vi "RM.set listbox size.vi"(8 "error in (no error)":errorcluster, 10 "Pane Refnum":refnum<vi>) -> (0 "error out":errorcluster)   [LabVIEW 2016, in "FPGA Resource Manager.lvlib"]
uses:
  FPGA Resource Manager.lvlib
  <vilib>/Utility/miscctls.llb/LVRowAndColumnTypeDef.ctl
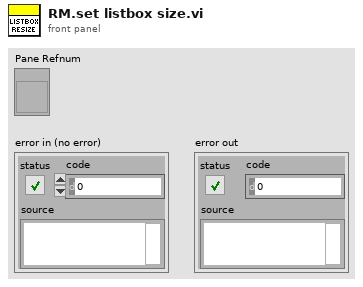
[diagram p1: front panel]
types:
  T1 = typedef "LVRowAndColumnTypeDef.ctl" = cluster{"Row":i32, "Column":i32}
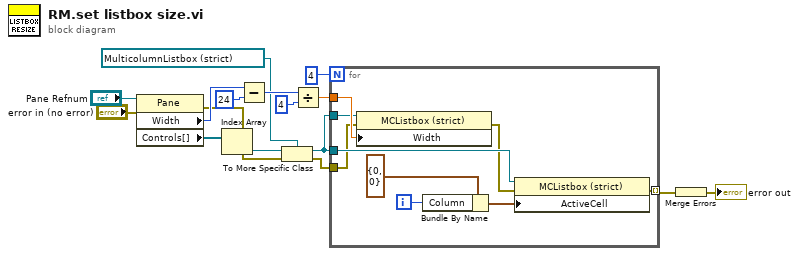
[diagram p0: block diagram]
diagram:
  n1 = property on="Property Node" class="Pane"(reference="Pane Refnum", error in="error in (no error)") -> (error out=w4:errorcluster, "Width"=w13:u32, "Controls[]"=w16:refnum<vi>[])  [unwired: 1 out]
  n2 = Index Array(array=w16) -> (element=w7:refnum<vi>)  [unwired: 1 in]
  n3 = Subtract(x=w13, y=u32 24) -> (x-y=w14:u32)
  n4 = To More Specific Class(target class=refnum<vi> refnum ("MulticolumnListbox in"), reference=w7, error in=w4) -> (specific class reference=w6:refnum<vi>, error out=w3:errorcluster)
  n5 = Divide(x=w14, y=u32 4) -> (x/y=w12:dbl)
  n6 = for {
    N: 4 -> [_]
    tunnel: w12 -> [w22]
    tunnel: w6 -> [w21]
    tunnel: w6 -> [w20]
    tunnel: w3 -> [w19]
    tunnel: [w17] -> w2 mode=indexing
    i -> [w24]
    n7 = property on="Property Node" class="MCListbox (strict)"(reference=w20, error in=w19, "Width"=w22) -> (error out=w18:errorcluster)  [unwired: 1 out]
    n8 = Bundle By Name(cluster=T1 {"Row"=0, "Column"=0} ("Active Cell:Active Cell"), "Column"=w24) -> (w23:T1)
    n9 = property on="Property Node" class="MCListbox (strict)"(reference=w21, error in=w18, "ActiveCell"=w23) -> (error out=w17:errorcluster)  [unwired: 1 out]
  }
  n10 = Merge Errors(w2) -> (→"error out":errorcluster)
